vi "FL_Calculate_Coordinates_for_saving.vi"(3 "Magnets coords in":T1) -> (1 "Output cluster of data":T2)   [LabVIEW 2018, in "Tracker.lvlib"]
uses:
  Tracker.lvlib
panel:
  out "Error Out":errorcluster
  in  "Error In":errorcluster
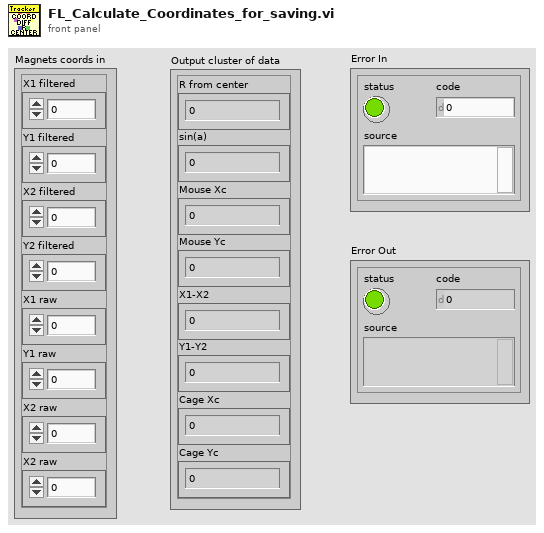
[diagram p1: front panel]
types:
  T1 = cluster{"X1 filtered":dbl, "Y1 filtered":dbl, "X2 filtered":dbl, "Y2 filtered":dbl, "X1 raw":dbl, "Y1 raw":dbl, "X2 raw":dbl, "X2 raw":dbl}
  T2 = cluster{"R from center":dbl, "sin(a)":dbl, "Mouse Xc":dbl, "Mouse Yc":dbl, "X1-X2":dbl, "Y1-Y2":dbl, "Cage Xc":dbl, "Cage Yc":dbl}
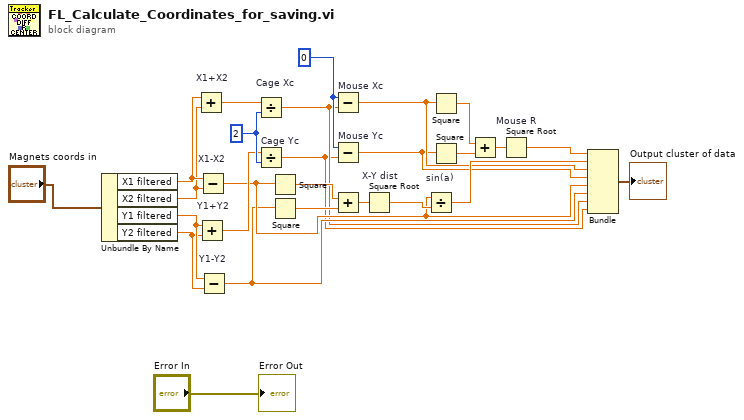
[diagram p0: block diagram]
diagram:
  w16 = 0
  w19 = 2
  n1 = Unbundle By Name("Magnets coords in") -> ("X1 filtered"=w15:dbl, "X2 filtered"=w14:dbl, "Y1 filtered"=w13:dbl, "Y2 filtered"=w12:dbl)
  n2 = Add "X1+X2"(x=w15, y=w14) -> (x+y=w17:dbl)
  n3 = Add "Y1+Y2"(x=w13, y=w12) -> (x+y=w18:dbl)
  n4 = Subtract "X1-X2"(x=w15, y=w14) -> (x-y=w7:dbl)
  n5 = Subtract "Y1-Y2"(x=w13, y=w12) -> (x-y=w6:dbl)
  n6 = Divide "Cage Xc"(x=w17, y=w19) -> (x/y=w5:dbl)
  n7 = Divide "Cage Yc"(x=w18, y=w19) -> (x/y=w4:dbl)
  n8 = Square(x=w7) -> (x^2=w20:dbl)
  n9 = Square(x=w6) -> (x^2=w21:dbl)
  n10 = Subtract "Mouse Xc"(x=w16, y=w5) -> (x-y=w9:dbl)
  n11 = Subtract "Mouse Yc"(x=w16, y=w4) -> (x-y=w8:dbl)
  n12 = Add(x=w20, y=w21) -> (x+y=w22:dbl)
  n13 = Square Root "X-Y dist"(x=w22) -> (sqrt(x)=w23:dbl)
  n14 = Divide "sin(a)"(x=w7, y=w23) -> (x/y=w10:dbl)
  n15 = Square(x=w9) -> (x^2=w24:dbl)
  n16 = Square(x=w8) -> (x^2=w25:dbl)
  n17 = Add(x=w24, y=w25) -> (x+y=w26:dbl)
  n18 = Square Root "Mouse R"(x=w26) -> (sqrt(x)=w11:dbl)
  n19 = Bundle(w11, w10, w9, w8, w7, w6, w5, w4) -> (→"Output cluster of data":cluster{dbl, dbl, dbl, dbl, dbl, dbl, dbl, dbl})  [unwired: 1 in]
  "Error Out" <- "Error In"
